vi "Fetch Repo Details.vi"(8 "error in (no error)":errorcluster, 11 "Repo URL":string="http://download.ni.com/evaluation/labview/lvtn/vipm/") -> (0 "error out":errorcluster, 3 "Repo out":refnum<class "Repo.lvclass">)   [LabVIEW 2016, in "Packages.lvlib" / "VIPM.lvlib"]
uses:
  VIPM.lvlib
  Repo_class/Repo.lvclass
  Repo_class/RepoType--enum.ctl
  Repo_class/Repo.lvclass/Repo.ctl
  Repo_class/Write URL.vi
  Repo_class/Write RepoType.vi
  <vilib>/httpClient/LabVIEWHTTPClient.lvlib
  WSsupport/WSsupport.lvlib
  <vilib>/zip/NI_Unzip.lvlib
  <vilib>/Utility/config.llb/NI_LVConfig.lvlib
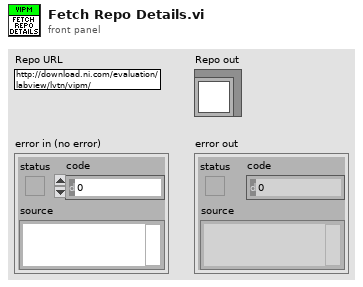
[diagram p1: front panel]
types:
  T1 = typedef "Packages.lvlib/Repo.lvclass/RepoType--enum.ctl" = enum16{"VIPM", "NIPM", "GPM"}
  T2 = typedef "NI_LVConfig.lvlib/Config Data RefNum.ctl" = refnum<k1>
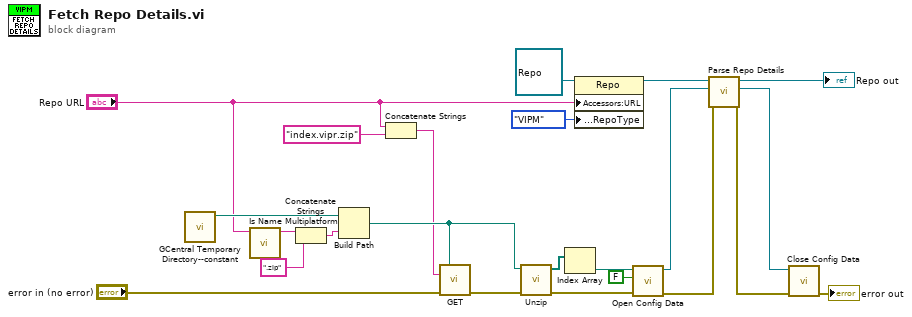
[diagram p0: block diagram]
diagram:
  n1 = call "GCentral Temporary Directory--constant.vi"() -> ("GCentral Temporary Directory"=w8:path)  [unwired: 11 in]
  n2 = call <vilib>:"Is Name Multiplatform.vi"("filename"="Repo URL") -> ("suggested filename"=w6:string)  [unwired: 6 in, 4 out]
  n3 = Concatenate Strings(w6, ".zip" ("string")) -> (w5:string)
  n4 = Build Path(base path=w8, name or relative path=w5) -> (appended path=w21:path)
  n5 = Concatenate Strings("Repo URL", "index.vipr.zip" ("string")) -> (w17:string)
  n6 = call <vilib>:"GET.vi"("output file"=w21, "url"=w17, "error in (no error)"="error in (no error)") -> ("error out"=w22:errorcluster)  [unwired: 9 in, 3 out]
  n7 = call <vilib>:"Unzip.vi"("error in (no error)"=w22, "Zip file"=w21) -> ("error out"=w19:errorcluster, "Unzipped files"=w20:path[])  [unwired: 7 in, 1 out]
  n8 = Index Array(array=w20) -> (element=w16:path)  [unwired: 1 in]
  n9 = property class="Repo"(reference=refnum<class "Repo.lvclass"> refnum ("Packages.lvlib:Repo"), "Accessors:URL"="Repo URL", "Accessors:RepoType"=RepoType--enum."VIPM" ("RepoType")) -> (reference out=w10:refnum<class "Repo.lvclass">)  [unwired: 1 in, 1 out]
  n10 = call <vilib>:"Open Config Data.vi"("error in (no error)"=w19, "create file if necessary (T)"=FALSE, "configuration file path"=w16) -> ("error out"=w13:errorcluster, "refnum"=w14:T2)  [unwired: 6 in, 1 out]
  n11 = call "Parse Repo Details.vi"("error in (no error)"=w13, "Repo file in"=w14, "Repo in"=w10) -> ("error out"=w11:errorcluster, "Repo file out"=w3:T2, "Repo out"=→"Repo out":refnum<class "Repo.lvclass">)  [unwired: 6 in]
  n12 = call <vilib>:"Close Config Data.vi"("error in (no error)"=w11, "refnum"=w3) -> ("error out"=→"error out":errorcluster)  [unwired: 8 in, 1 out]
